vi "BasicPath.xio.vi"() -> (0 "stripped path":path)   [LabVIEW 2018]
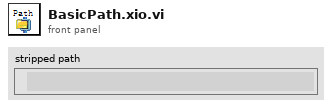
[diagram p1: front panel]
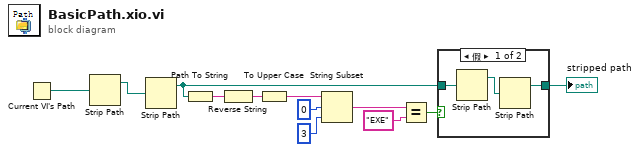
[diagram p0: block diagram]
diagram:
  n1 = Current VI's Path() -> (path=w1:path)
  n2 = Strip Path(path=w1) -> (stripped path=w2:path)  [unwired: 1 out]
  n3 = Strip Path(path=w2) -> (stripped path=w4:path)  [unwired: 1 out]
  n4 = Path To String(path=w4) -> (string=w12:string)
  n5 = Reverse String(1:w12) -> (0:w11:string)
  n6 = To Upper Case(1:w11) -> (0:w10:string)
  n7 = String Subset(string=w10, offset (0)=0 ("偏移量(0)"), length (rest)=3 ("长度（剩余）")) -> (substring=w7:string)
  n8 = Equal?(x=w7, y="EXE") -> (x = y?=w5:bool)
  n9 = case shown="假" w5 {
    tunnel: w4 -> [w15 w16]
    tunnel: [w13 w16] -> w3
    frame False {
      n10 = Strip Path(path=w15) -> (stripped path=w14:path)  [unwired: 1 out]
      n11 = Strip Path(path=w14) -> (stripped path=w13:path)  [unwired: 1 out]
    }
    frame True {
    }
  }
  "stripped path" <- w3
